vi "Start continous acquisition.vi"(5 "N samples":i32, 7 "Samples":enum16{"Single", "Multiple"}(ring), 8 "error in":errorcluster, 9 "Timeout":i32, 10 "Task list":T1, 11 "Module ID":i32=-1) -> (0 "error out":errorcluster)   [LabVIEW 2020, in "NI DAQ.lvlib"]
doc: "Request to acquire continuously from DAQ device with a predefined Timeout period.\n_____\nCreated using DQMH Event Scripter 6.1.0.128."
uses:
  NI DAQ.lvlib
  Support/Task list.ctl
  Start continous acquisition Argument--cluster.ctl
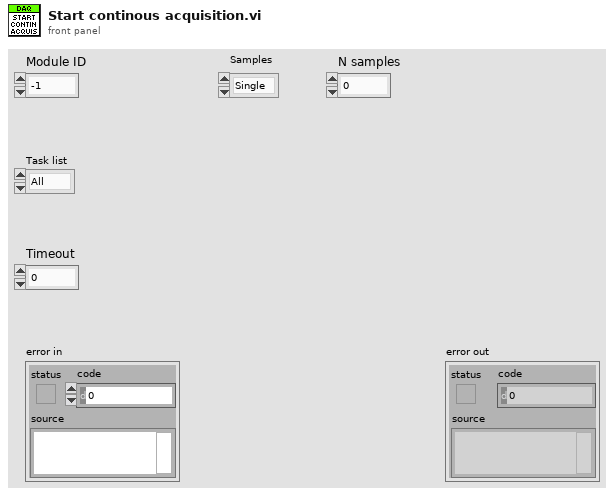
[diagram p1: front panel]
types:
  T1 = typedef "NI DAQ.lvlib/Task list.ctl" = enum16{"All", "DO task", "DI task", "AO task", "AI task"}
  T2 = typedef "NI DAQ.lvlib/Start continous acquisition Argument--cluster.ctl" = cluster{"Module ID":i32, "Task list":T1, "Timeout":i32, "Acq type":enum16{"Single", "Multiple"}, "N samples":i32, "Data in":variant}
  T3 = typedef "NI DAQ.lvlib/Request Events--cluster.ctl" = cluster{"Stop Module":refnum<user-event>, "Show Panel":refnum<user-event>, "Hide Panel":refnum<user-event>, "Show Diagram":refnum<user-event>, "Get Module Execution Status":refnum<user-event>, "Set device ID":refnum<user-event>, "Get channel list":refnum<user-event>, "Create DO task":refnum<user-event>, "Start task":refnum<user-event>, "Stop task":refnum<user-event>, "Write DO":refnum<user-event>, "Create DI channel":refnum<user-event>, "Read DI":refnum<user-event>, "Get task ref":refnum<user-event>, "Wake up HL":refnum<user-event>, "Sleep HL":refnum<user-event>, "Create AI channel":refnum<user-event>, "Read AI":refnum<user-event>, "Create AO channel":refnum<user-event>, "Write AO":refnum<user-event>, "Validate connection":refnum<user-event>, "Start continous acquisition":refnum<user-event>, "Stop continuous acquisition":refnum<user-event>}
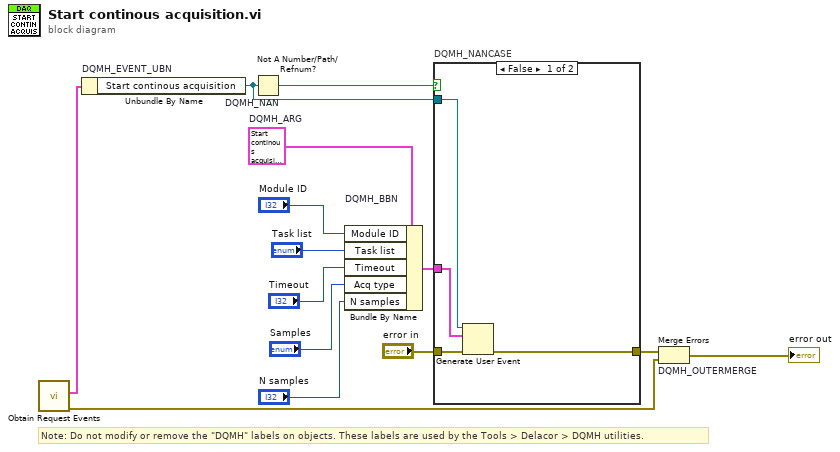
[diagram p0: block diagram]
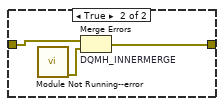
[diagram p2: hidden frame]
diagram:
  w8 = T2 {"Module ID"=-1, "Task list"=enum."All", "Timeout"=0, "Acq type"=enum."Single", "N samples"=0, "Data in"=variant}  # DQMH_ARG
  # "Note: Do not modify or remove the \"DQMH\" labels on objects. These labels are used by the Tools > Delacor > DQMH utilities."
  n1 = call "Obtain Request Events.vi"() -> ("error out"=w2:errorcluster, "NI DAQ Request Events"=w1:T3)  [unwired: 10 in]
  n2 = Unbundle By Name "DQMH_EVENT_UBN"(w1) -> ("Start continous acquisition"=w10:refnum<user-event>)
  n3 = Not A Number/Path/Refnum? "DQMH_NAN"(number/path/refnum=w10) -> (NaN/Path/Refnum?=w11:bool)
  n4 = Bundle By Name "DQMH_BBN"(cluster=w8, "Module ID"="Module ID", "Task list"="Task list", "Timeout"="Timeout", "Acq type"="Samples", "N samples"="N samples") -> (w12:T2)
  n5 = case "DQMH_NANCASE" shown="False" w11 {
    tunnel: "error in" -> [w18 w21]
    tunnel: [w17 w20] -> w9
    tunnel: w10 -> [w16 _]
    tunnel: w12 -> [w15 _]
    frame False {
      n6 = Generate User Event(user event=w16, event data cluster=w15, error in=w18) -> (error out=w17:errorcluster)  [unwired: 1 in, 1 out]
    }
    frame True {
      n7 = call "Module Not Running--error.vi"() -> ("error out"=w19:errorcluster)  [unwired: 11 in]
      n8 = Merge Errors "DQMH_INNERMERGE"(w21, w19) -> (w20:errorcluster)
    }
  }
  n9 = Merge Errors "DQMH_OUTERMERGE"(w9, w2) -> (→"error out":errorcluster)
